vi "Channel Index by Name.vi"(8 "error in (no error)":errorcluster, 10 "Channel Name":string, 11 "CIFCorePlugin in":refnum<class "CIFCorePlugin.lvclass">) -> (0 "error out":errorcluster, 2 "Channel Index":i32=65535, 3 "CIFCorePlugin out":refnum<class "CIFCorePlugin.lvclass">)   [LabVIEW 2021, in "CIFCorePlugin.lvclass"]
uses:
  CIFCorePlugin.lvclass
  Channels/CIFChannelMng/CIFChannelMng.lvclass
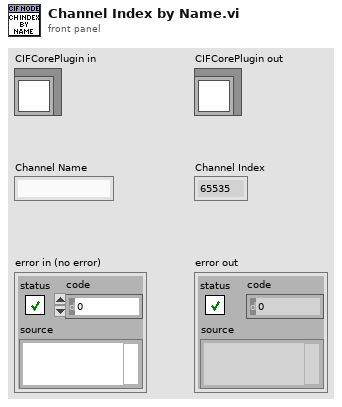
[diagram p1: front panel]
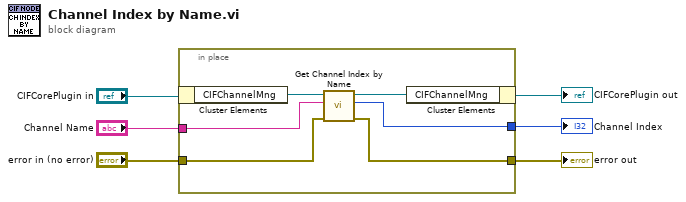
[diagram p0: block diagram]
diagram:
  n1 = in-place {
    in-place-border: "error in (no error)" -> [w10]
    in-place-border: [w9] -> w5
    in-place-border: "Channel Name" -> [w8]
    in-place-border: [w7] -> w1
    n2 = in-place-cluster #1("CIFCorePlugin in") -> ("CIFChannelMng"=w12:refnum<class "CIFChannelMng.lvclass">)
    n3 = call "Get Channel Index by Name.vi"("error in (no error)"=w10, "Channel Name"=w8, "CIFChannelMng in"=w12) -> ("error out"=w9:errorcluster, "Channel Index"=w7:i32, "CIFChannelMng out"=w11:refnum<class "CIFChannelMng.lvclass">)  [unwired: 6 in]
    n4 = in-place-cluster #1("CIFChannelMng"=w11) -> (→"CIFCorePlugin out":refnum<class "CIFCorePlugin.lvclass">)
  }
  "error out" <- w5
  "Channel Index" <- w1
